vi "Apply special move.vi"(8 "error in (no error)":errorcluster, 10 "Position in":refnum<class "Position.lvclass">, 11 "CastleRestricting in":refnum<class "CastleRestricting.lvclass">) -> (0 "error out":errorcluster, 2 "Position out":refnum<class "Position.lvclass">, 3 "CastleRestricting out":refnum<class "CastleRestricting.lvclass">)   [LabVIEW 2016, in "Chesslib.lvlib" / "CastleRestricting.lvclass"]
uses:
  CastleRestricting.lvclass
  Position/Position.lvclass
  CastleRestricting.lvclass/CastleRestricting.ctl
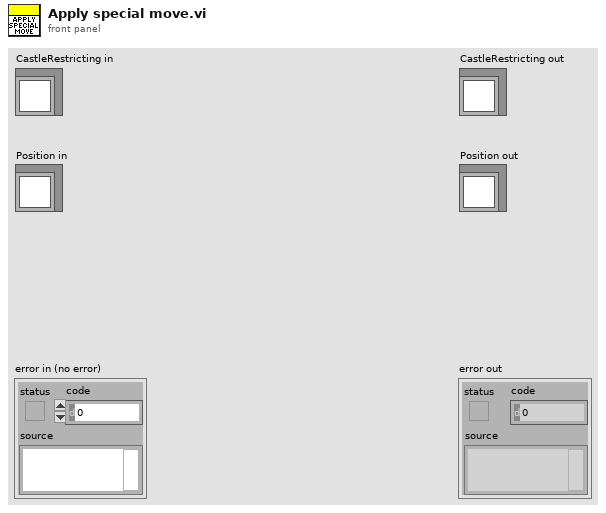
[diagram p1: front panel]
types:
  T1 = typedef "Chesslib.lvlib/Color.ctl" = enum16{"Light", "Dark"}
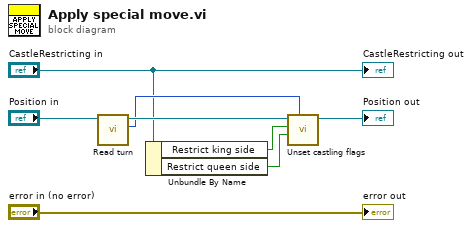
[diagram p0: block diagram]
diagram:
  n1 = call "Read turn.vi"("Position in"="Position in") -> ("Turn"=w4:T1, "Position out"=w6:refnum<class "Position.lvclass">)  [unwired: 9 in]
  n2 = Unbundle By Name("CastleRestricting in") -> ("Restrict king side"=w2:bool, "Restrict queen side"=w1:bool)
  n3 = call "Unset castling flags.vi"("Color"=w4, "Unflag queen side (F)"=w1, "Unflag king side (F)"=w2, "Position in"=w6) -> ("Position out"=→"Position out":refnum<class "Position.lvclass">)  [unwired: 6 in, 1 out]
  "error out" <- "error in (no error)"
  "CastleRestricting out" <- "CastleRestricting in"
